vi "Identities.vi"(8 "error in (no error)":errorcluster, 11 "LoggingAPI in":refnum<class "LoggingAPI.lvclass">) -> (0 "error out":errorcluster, 2 "Identities":refnum<class "Identity.lvclass">[](array[class]), 3 "LoggingAPI out":refnum<class "LoggingAPI.lvclass">)   [LabVIEW 2020, in "VolatusData.lvlib" / "LoggingAPI.lvclass"]
uses:
  LoggingAPI.lvclass
  LoggingIdentity/LoggingIdentity.lvclass
  C:/dev/lv20CE/relink/lv-volatus/Volatus/LoggingIdentity/LoggingIdentity.lvclass
  C:/dev/lv20CE/relink/lv-volatus/Volatus/Identity/Identity.lvclass
  Volatus/Identity/Identity.lvclass
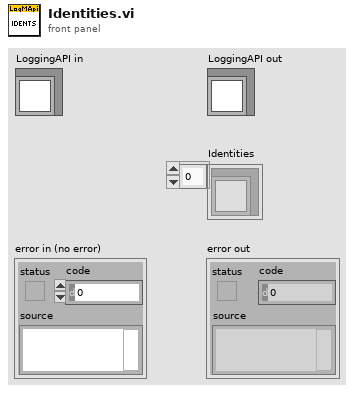
[diagram p1: front panel]
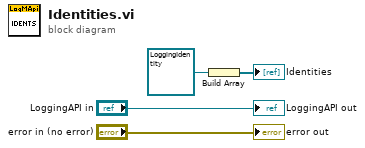
[diagram p0: block diagram]
diagram:
  n1 = Build Array(refnum<class "LoggingIdentity.lvclass"> refnum ("VolatusDataLogger:LoggingIdentity.lvclass")) -> (→"Identities":refnum<class "LoggingIdentity.lvclass">[])
  "error out" <- "error in (no error)"
  "LoggingAPI out" <- "LoggingAPI in"
